vi "VisualizeSiemens.vi"() -> ()   [LabVIEW 2018, in "Visualization.lvlib" / "VisualizeSensor.lvclass"]
doc: "This VI listens for any measurement data associated with the provided PluginName and displays it to the user for analysis. The display is only suitable for data coming from the Siemens Plugin."
uses:
  VisualizeSensor.lvclass
  Sensor/SensorShared/clSensorData.ctl
  <extravilib>/ChannelInstances/Tag-bool/Read With Abort.vi
  <extravilib>/ChannelInstances/Tag-bool/Write With Abort.vi
  <extravilib>/ChannelInstances/Tag-bool/Instantiate.vi
  <extravilib>/ChannelInstances/Tag-bool/EndpointRead.vi
  <vilib>/Utility/error.llb/Error Cluster From Error Code.vi
  <extravilib>/ChannelInstances/Tag-bool/Endpoint.vi
  <vilib>/ErrorRing/Error Ring.xnode
  <userlib>/NIST/NISTErrorLib/NISTErrorLib.lvlib
  VisualizeBase/VisualizeBase_class/VisualizeBase.lvclass
  Sensor/SensorShared/SensorShared.lvlib
  Sensor/SensorModule/SensorModule.lvlib
  <extravilib>/ChannelInstances/Tag-bool.lvlib
panel:
  out "String Results":string[](array[string])
  in  "Tab Control":enum32{"Chart"}(tab)
  out "Siemens":waveform(dbl)[](graph)=[{"t0"=timestamp(3657200531.6397257 s since 1904-01-01), "dt"=1.0, "Y"=[46.19]}, {"t0"=timestamp(3657200531.6397257 s since 1904-01-01), "dt"=1.0, "Y"=[2.0]}, {"t0"=timestamp(3657200531.6397257 s since 1904-01-01), "dt"=1.0, "Y"=[60.0]}]
  in  "PlotYAxis":u32[](array[numeric])=[0, 1, 0] max=1
  out "Incorrect DataType?":bool
  out "ErrorArray":errorcluster[](array[cluster])
  in  "PluginName":string="Sensor.SiemensDEM0"
  in  "btnStop":bool
  in  "btnReset":bool
  in  "btnClear":bool
  # "0=Left Axis and 1=Right Axis"
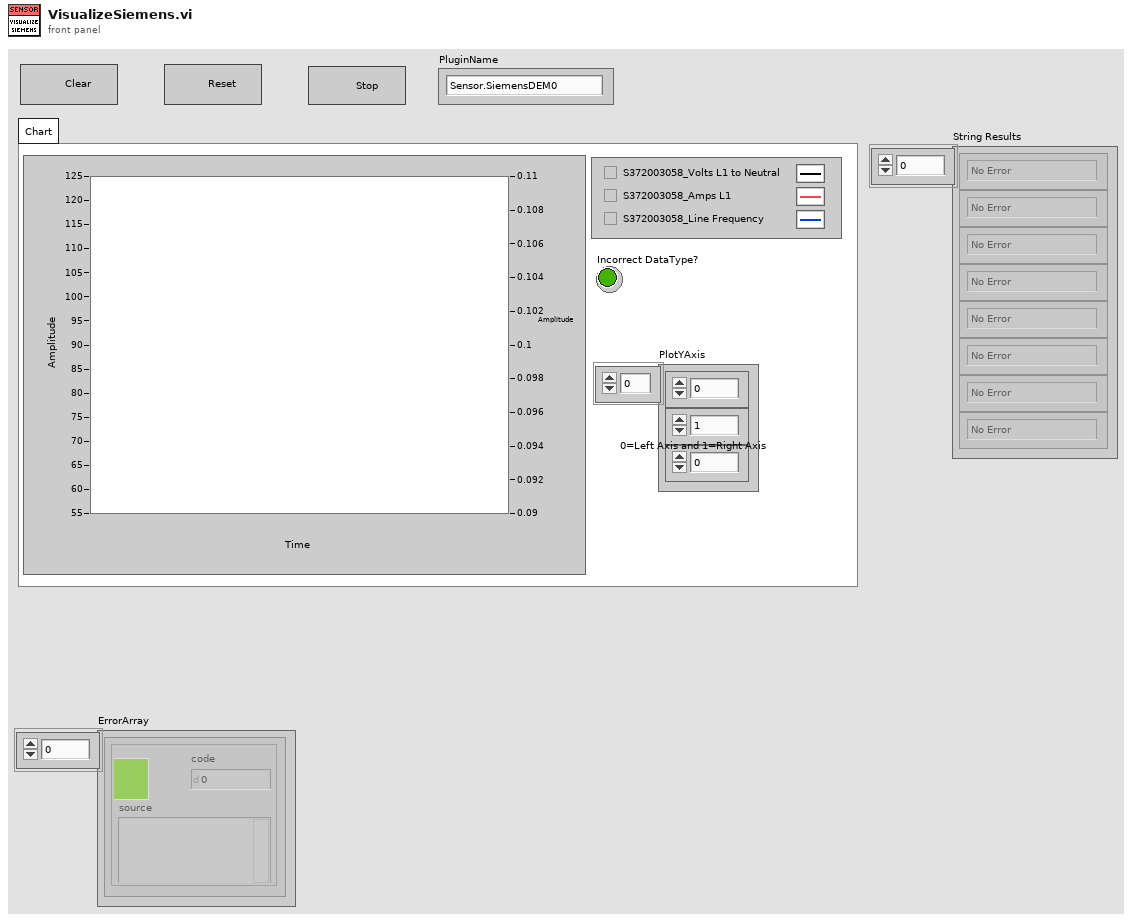
[diagram p1: front panel]
types:
  T1 = typedef "Visualization.lvlib/VisualizeBase.lvclass/clRequestEvents.ctl" = cluster{"StopRequest":refnum<user-event>, "ResetRequest":refnum<user-event>}
  T2 = typedef "SensorShared.lvlib/clBroadcastEvents.ctl" = cluster{"DidInit":refnum<user-event>, "StatusUpdate":refnum<user-event>, "ErrorReport":refnum<user-event>, "DidStop":refnum<user-event>, "PathToINI":refnum<user-event>, "SensorReport":refnum<user-event>, "SensorConfig":refnum<user-event>}
  T3 = typedef "SensorShared.lvlib/clSensorData.ctl" = cluster{"SensorType":string, "SensorData":variant}
  T4 = typedef "Tag-bool.lvlib/))Channel.ctl" = refnum<queue>
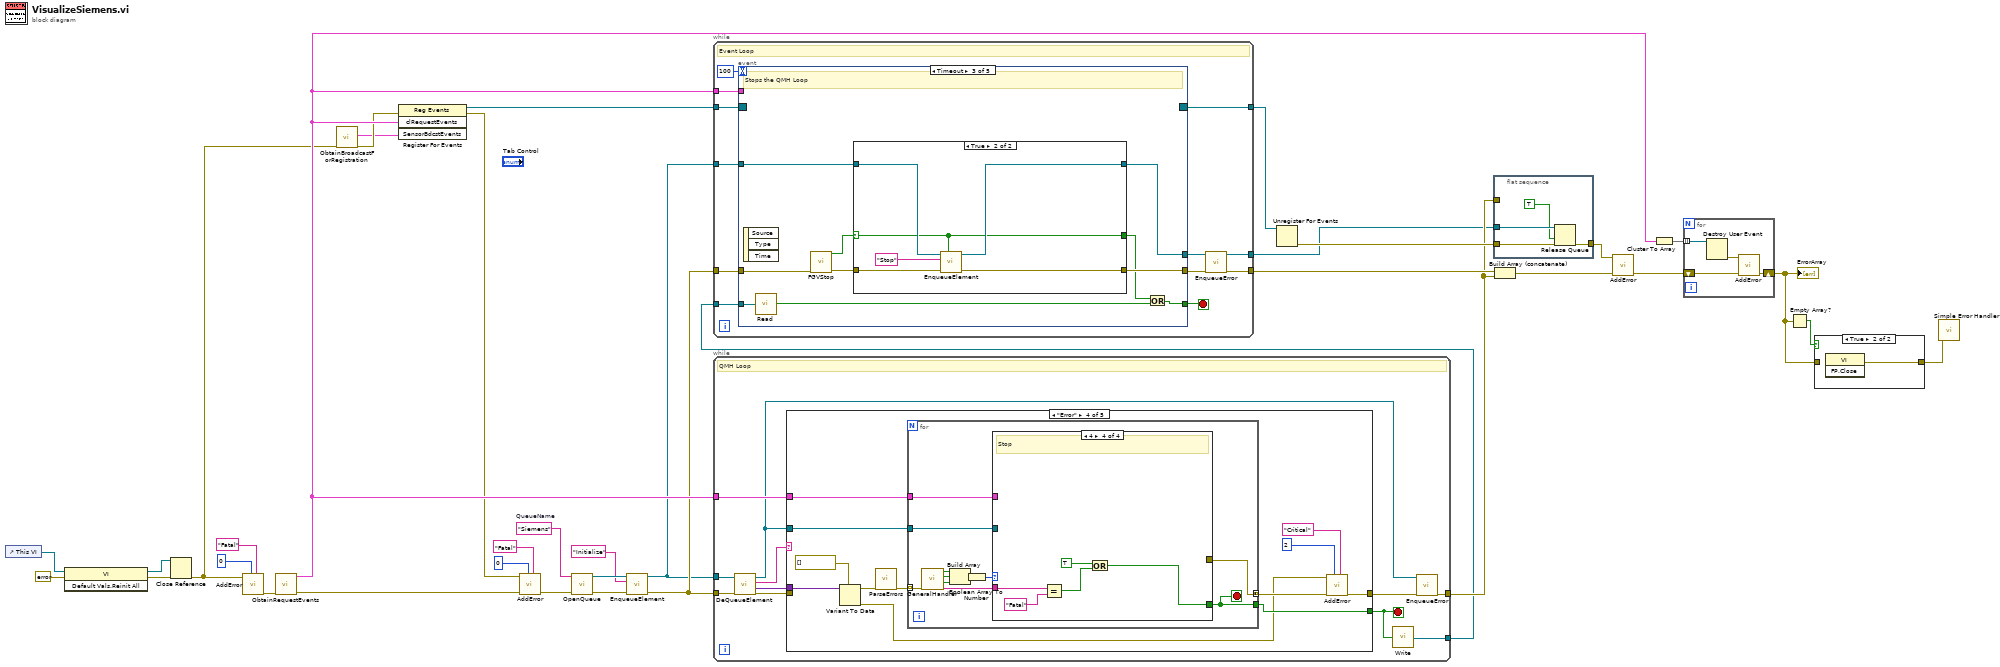
[diagram p0: block diagram]
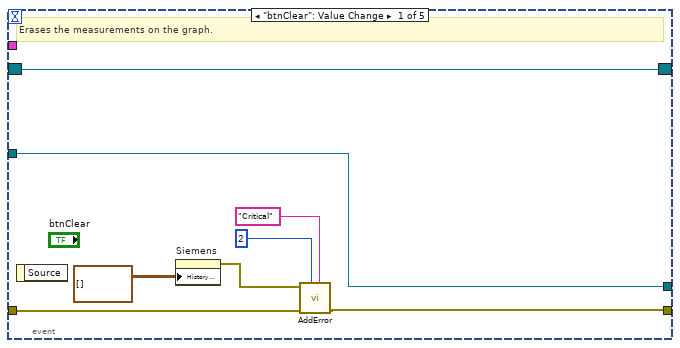
[diagram p2: hidden frame]
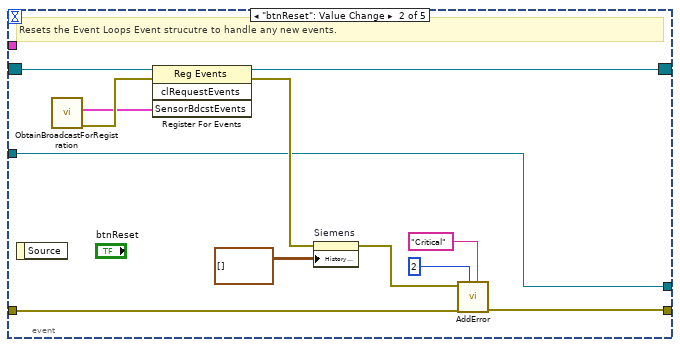
[diagram p3: hidden frame]
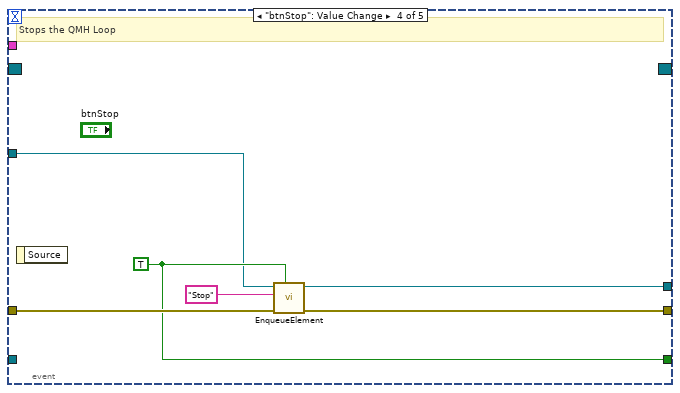
[diagram p5: hidden frame]
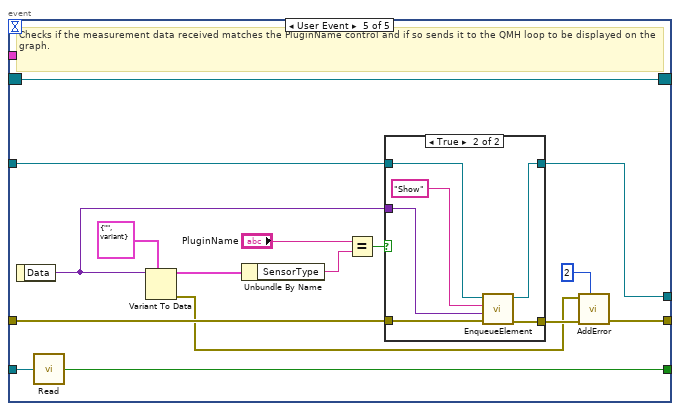
[diagram p6: hidden frame]
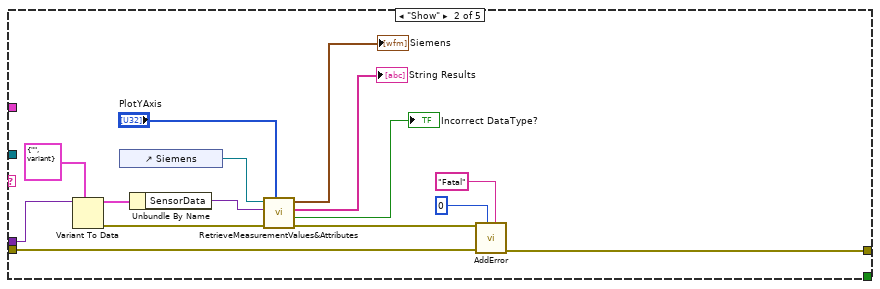
[diagram p9: hidden frame]
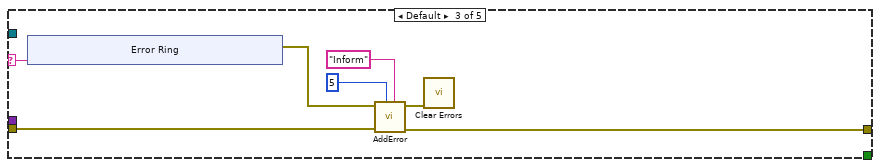
[diagram p10: hidden frame]
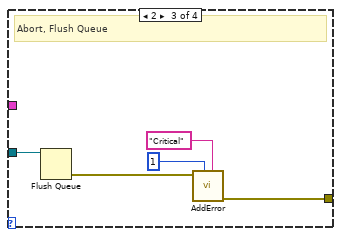
[diagram p13: hidden frame]
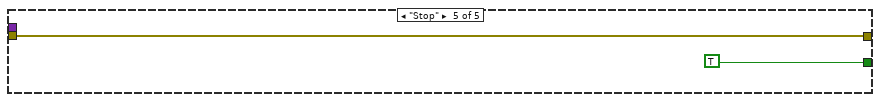
[diagram p14: hidden frame]
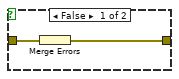
[diagram p15: hidden frame]
diagram:
  w11 = "Siemens"  # QueueName
  n1 = control-ref of="This VI"() -> (w25:refnum<vi>)
  n2 = invoke class="VI" method="Default Vals.Reinit All"(reference=w25, error in=errorcluster {"status"=FALSE, "code"=0, "source"=""} ("error in (no error)")) -> (reference out=w22:refnum<vi>, error out=w23:errorcluster)  [unwired: 1 in, 1 out]
  n3 = Close Reference(reference=w22, error in (no error)=w23) -> (error out=w13:errorcluster)
  n4 = call <userlib>:"AddError.vi"("Severity"="Fatal", "Priority"=u8 0, "error in (no error)"=w13) -> ("ErrorArray Out"=w35:errorcluster[])  [unwired: 7 in, 1 out]
  n5 = call "ObtainRequestEvents.vi"("Error"=w35) -> ("Error"=w20:errorcluster[], "clRequestEvents"=w27:T1)  [unwired: 9 in]
  n6 = call "ObtainBroadcastForRegistration.vi"("error in (no error)"=w13) -> ("error out"=w14:errorcluster, "SensorBdcstEvents"=w2:T2)  [unwired: 9 in]
  n7 = register-events(error in=w14, w27, w2) -> (reference out=w36:refnum<event-registration>, error out=w18:errorcluster)  [unwired: 1 in]
  n8 = call <userlib>:"AddError.vi"("Severity"="Fatal", "Priority"=u8 0, "ErrorArray In"=w20, "error in (no error)"=w18) -> ("ErrorArray Out"=w12:errorcluster[])  [unwired: 6 in, 1 out]
  n9 = call "OpenQueue.vi"("Error Array In"=w12, "QueueName"=w11) -> ("Error Array Out"=w9:errorcluster[], "queue out"=w10:refnum<queue>)  [unwired: 8 in]
  n10 = call "EnqueueElement.vi"("Error Array In"=w9, "Message"="Initialize", "queue in"=w10) -> ("Error Array Out"=w7:errorcluster[], "queue out"=w6:refnum<queue>)  [unwired: 7 in]
  n11 = while {
    tunnel: w7 -> [w41]
    tunnel: [w44] -> w15
    tunnel: w6 -> [w40]
    tunnel: w27 -> [w46]
    tunnel: [w37] -> w1
    stop <- w47 stop-if-true
    # "QMH Loop"
    n12 = call "DeQueueElement.vi"("Error Array In"=w41, "Queue In"=w40) -> ("Error Array Out"=w39:errorcluster[], "Data"=w42:variant, "Message"=w43:string, "Queue Out"=w38:refnum<queue>)  [unwired: 6 in]
    n13 = case shown="\"Error\"" w43 {
      selector: w43 -> [_ _ w70 _ _]
      tunnel: w42 -> [_ w55 _ w89 _]
      tunnel: w39 -> [w48 w61 w68 _ w111]
      tunnel: [w48 w63 w67 w79 w111] -> w45
      tunnel: [_ _ _ w85 TRUE] -> w47
      tunnel: w46 -> [_ _ _ w84 _]
      tunnel: w38 -> [_ _ _ w83 _]
      frame "Initialize" {
      }
      frame "Show" {
        n14 = Variant To Data(type=T3 {"SensorType"="", "SensorData"=variant} ("clSensorData"), Variant=w55) -> (data=w53:T3, error out=w54:errorcluster)  [unwired: 1 in]
        n15 = control-ref of="Siemens"() -> (w62:refnum<vi>)
        n16 = Unbundle By Name(w53) -> ("SensorData"=w50:variant)
        n17 = call "RetrieveMeasurementValues&Attributes.vi"("PlotYScale"="PlotYAxis", "error in (no error)"=w54, "Variant"=w50, "WaveformChartReference"=w62) -> ("error out"=w57:errorcluster, "Incorrect DataType?"=→"Incorrect DataType?":bool, "Array Of Strings"=→"String Results":string[], "WaveformArrayOut"=→"Siemens":waveform(dbl)[])  [unwired: 3 in, 1 out]
        n18 = call <userlib>:"AddError.vi"("Severity"="Fatal" ("String"), "Priority"=u8 0, "ErrorArray In"=w61, "error in (no error)"=w57) -> ("ErrorArray Out"=w63:errorcluster[])  [unwired: 6 in, 1 out]
      }
      frame Default {
        n19 = xnode "Error Ring"("parameter 0"=w70) -> ("error out"=w69:errorcluster)
        n20 = call <userlib>:"AddError.vi"("Severity"="Inform" ("String"), "Priority"=u8 5, "ErrorArray In"=w68, "error in (no error)"=w69) -> ("ErrorArray Out"=w67:errorcluster[], "error out"=w66:errorcluster)  [unwired: 6 in]
        n21 = call <vilib>:"Clear Errors.vi"("error in (no error)"=w66) -> ()  [unwired: 5 in, 2 out]
      }
      frame "Error" {
        n22 = Variant To Data(type=errorcluster[] [], Variant=w89) -> (data=w87:errorcluster[], error out=w78:errorcluster)  [unwired: 1 in]
        n23 = call <userlib>:"ParseErrors.vi"("ErrorArray"=w87) -> ("ErrorArray"=w86:errorcluster[])  [unwired: 8 in, 2 out]
        n24 = for {
          tunnel: w86 -> [w100] mode=indexing
          tunnel: [w94] -> w80 mode=concatenating
          tunnel: [w92] -> w85
          tunnel: w84 -> [w91]
          tunnel: w83 -> [w90]
          stop <- w92 stop-if-true
          n25 = call <userlib>:"GeneralHandler.vi"("error in (no error)"=w100) -> ("Severity"=w93:string, "Stop"=w97:bool, "Abort"=w98:bool, "Continue"=w99:bool)  [unwired: 6 in, 1 out]
          n26 = Build Array(w99, w98, w97) -> (w96:bool[])
          n27 = Boolean Array To Number(Boolean array=w96) -> (number=w95:u32)
          n28 = case shown="4" w95 {
            tunnel: [_ _ w105 _] -> w94
            tunnel: w93 -> [_ _ _ w110]
            tunnel: [_ _ _ w106] -> w92
            tunnel: w91 -> [_ _ _ _]
            tunnel: w90 -> [_ _ w101 _]
            frame 0, Default {
              # "No Dialog"
            }
            frame 1 {
              # "Continue"
            }
            frame 2 {
              # "Abort, Flush Queue"
              n29 = Flush Queue(queue=w101) -> (error out=w104:errorcluster)  [unwired: 1 in, 2 out]
              n30 = call <userlib>:"AddError.vi"("Severity"="Critical" ("String"), "Priority"=u8 1, "error in (no error)"=w104) -> ("ErrorArray Out"=w105:errorcluster[])  [unwired: 7 in, 1 out]
            }
            frame 4 {
              # "Stop"
              n31 = Equal?(x=w110, y="Fatal" ("x")) -> (x = y?=w107:bool)
              n32 = Or(x=TRUE, y=w107) -> (x .or. y?=w106:bool)
            }
          }
        }
        n33 = call <userlib>:"AddError.vi"("Severity"="Critical", "Priority"=u8 2, "ErrorArray In"=w80, "error in (no error)"=w78) -> ("ErrorArray Out"=w79:errorcluster[])  [unwired: 6 in, 1 out]
      }
      frame "Stop" {
      }
    }
    n34 = call <extravilib>:"Write.vi"("element"=w47) -> ("channel"=w37:T4)  [unwired: 1 out]
    n35 = call "EnqueueError.vi"("Error Array In"=w45, "Queue in"=w38) -> ("Error Array Out"=w44:errorcluster[])  [unwired: 8 in, 1 out]
  }
  n36 = while {
    tunnel: w36 -> [w124]
    tunnel: [w118] -> w32
    tunnel: [w122] -> w34
    tunnel: w27 -> [w121]
    tunnel: w7 -> [w120]
    tunnel: w6 -> [w119]
    tunnel: [w115] -> w5
    tunnel: w1 -> [w113]
    stop <- w123 stop-if-true
    # "Event Loop"
    n37 = event shown="[2] Timeout" {
      selector: w124 -> [w126 w144 _ _ w180]
      dyn-events: [w126 w143 _ _ w180] -> w122
      timeout: 100 -> [_ _ _ _ _]
      tunnel: [_ _ w148 w166 w170] -> w123
      tunnel: [w129 w141 w150 w168 w183] -> w117
      tunnel: w121 -> [_ _ _ _ _]
      tunnel: w120 -> [w130 w142 w151 w169 w184]
      tunnel: w119 -> [w125 w134 w147 w164 w185]
      tunnel: [w125 w134 w146 w167 w181] -> w116
      tunnel: w113 -> [_ _ w154 _ w171]
      event "btnClear": Value Change {
        # "Erases the measurements on the graph."
        n38 = event-data() -> ()  [unwired: 1 in, 1 out]
        n39 = property on="Siemens" class="WFChart (strict)"("History Data"=waveform(dbl)[][] []) -> (error out=w128:errorcluster)  [unwired: 2 in, 1 out]
        n40 = call <userlib>:"AddError.vi"("Severity"="Critical", "Priority"=u8 2, "ErrorArray In"=w130, "error in (no error)"=w128) -> ("ErrorArray Out"=w129:errorcluster[])  [unwired: 6 in, 1 out]
      }
      event "btnReset": Value Change {
        # "Resets the Event Loops Event strucutre to handle any new events."
        n41 = event-data() -> ()  [unwired: 1 in, 1 out]
        n42 = call "ObtainBroadcastForRegistration.vi"() -> ("error out"=w135:errorcluster, "SensorBdcstEvents"=w133:T2)  [unwired: 10 in]
        n43 = register-events(reference=w144, error in=w135, w133) -> (reference out=w143:refnum<event-registration>, error out=w137:errorcluster)  [unwired: 1 in]
        n44 = property on="Siemens" class="WFChart (strict)"(error in=w137, "History Data"=waveform(dbl)[][] []) -> (error out=w136:errorcluster)  [unwired: 1 in, 1 out]
        n45 = call <userlib>:"AddError.vi"("Severity"="Critical", "Priority"=u8 2, "ErrorArray In"=w142, "error in (no error)"=w136) -> ("ErrorArray Out"=w141:errorcluster[])  [unwired: 6 in, 1 out]
      }
      event Timeout {
        # "Stops the QMH Loop"
        n46 = event-data() -> ()  [unwired: 1 in, 3 out]
        n47 = call <extravilib>:"Read.vi"("channel"=w154) -> ("element"=w149:bool)  [unwired: 1 in, 1 out]
        n48 = call "FGVStop.vi"("Error In"=w151) -> ("Error Out"=w152:errorcluster[], "Value"=w153:bool)  [unwired: 9 in]
        n49 = case shown="True" w153 {
          selector: w153 -> [w155 w158]
          tunnel: [w157 w161] -> w150
          tunnel: w152 -> [w157 w162]
          tunnel: w147 -> [w156 w160]
          tunnel: [w156 w159] -> w146
          tunnel: [w155 w158] -> w145
          frame False {
          }
          frame True {
            n50 = call "EnqueueElement.vi"("Priority? (F)"=w158, "Error Array In"=w162, "Message"="Stop", "queue in"=w160) -> ("Error Array Out"=w161:errorcluster[], "queue out"=w159:refnum<queue>)  [unwired: 6 in]
          }
        }
        n51 = Or(x=w145, y=w149) -> (x .or. y?=w148:bool)
      }
      event "btnStop": Value Change {
        w166 = TRUE ("Priority? (F)")
        # "Stops the QMH Loop"
        n52 = event-data() -> ()  [unwired: 1 in, 1 out]
        n53 = call "EnqueueElement.vi"("Priority? (F)"=w166, "Error Array In"=w169, "Message"="Stop", "queue in"=w164) -> ("Error Array Out"=w168:errorcluster[], "queue out"=w167:refnum<queue>)  [unwired: 6 in]
      }
      event User Event {
        # "Checks if the measurement data received matches the PluginName control and if so sends it to the QMH loop to be displayed on the graph."
        n54 = event-data() -> ("Data"=w177:variant)  [unwired: 1 in]
        n55 = call <extravilib>:"Read.vi"("channel"=w171) -> ("element"=w170:bool)  [unwired: 1 in, 1 out]
        n56 = Variant To Data(type=T3 {"SensorType"="", "SensorData"=variant} ("clSensorData"), Variant=w177) -> (data=w175:T3, error out=w176:errorcluster)  [unwired: 1 in]
        n57 = Unbundle By Name(w175) -> ("SensorType"=w174:string)
        n58 = Equal?(x="PluginName", y=w174) -> (x = y?=w172:bool)
        n59 = case shown="True" w172 {
          tunnel: [w186 w192] -> w182
          tunnel: w185 -> [w187 w191]
          tunnel: w184 -> [w186 w193]
          tunnel: [w187 w189] -> w181
          tunnel: w177 -> [_ w190]
          frame False {
          }
          frame True {
            n60 = call "EnqueueElement.vi"("Error Array In"=w193, "Data"=w190, "Message"="Show", "queue in"=w191) -> ("Error Array Out"=w192:errorcluster[], "queue out"=w189:refnum<queue>)  [unwired: 6 in]
          }
        }
        n61 = call <userlib>:"AddError.vi"("Priority"=u8 2, "ErrorArray In"=w182, "error in (no error)"=w176) -> ("ErrorArray Out"=w183:errorcluster[])  [unwired: 7 in, 1 out]
      }
    }
    n62 = call "EnqueueError.vi"("Error Array In"=w117, "Queue in"=w116) -> ("Error Array Out"=w118:errorcluster[], "Queue out"=w115:refnum<queue>)  [unwired: 8 in]
  }
  n63 = Unregister For Events(event registration refnum=w34) -> (error out=w31:errorcluster)  [unwired: 1 in]
  n64 = flat-sequence {
    tunnel: w31 -> [w197]
    tunnel: [w196] -> w29
    tunnel: w5 -> [w195]
    tunnel: w15 -> [_]
    frame #0 {
      n65 = Release Queue(queue=w195, force destroy? (F)=TRUE, error in (no error)=w197) -> (error out=w196:errorcluster)  [unwired: 2 out]
    }
  }
  n66 = Build Array (concatenate)(w32, w15) -> (w30:errorcluster[])
  n67 = call <userlib>:"AddError.vi"("ErrorArray In"=w30, "error in (no error)"=w29) -> ("ErrorArray Out"=w28:errorcluster[])  [unwired: 8 in, 1 out]
  n68 = Cluster To Array(cluster=w27) -> (array=w33:refnum<user-event>[])
  n69 = for {
    tunnel: w33 -> [w201] mode=indexing
    shift-right: [w200] -> w4
    shift-left: w28 -> [w199]
    n70 = Destroy User Event(user event=w201) -> (error out=w198:errorcluster)  [unwired: 1 in]
    n71 = call <userlib>:"AddError.vi"("ErrorArray In"=w199, "error in (no error)"=w198) -> ("ErrorArray Out"=w200:errorcluster[])  [unwired: 8 in, 1 out]
  }
  "ErrorArray" <- w4
  n72 = Empty Array?(array=w4) -> (empty?=w26:bool)
  n73 = case shown="True" w26 {
    tunnel: [w202 w204] -> w3
    tunnel: w4 -> [w203 _]
    frame False {
      n74 = Merge Errors(w203) -> (w202:errorcluster)
    }
    frame True {
      n75 = invoke class="VI" method="FP.Close"() -> (error out=w204:errorcluster)  [unwired: 3 in, 2 out]
    }
  }
  n76 = call <vilib>:"Simple Error Handler.vi"("error in (no error)"=w3) -> ()  [unwired: 4 in, 5 out]
